vi "LJM logger write register list config.vi"(9 "Register List":string[](array[string])=["DAC0", "DAC1"], 10 "Filename":string="LJM_Open_Any.cfg", 11 "Working Directory":path) -> (0 "error out":errorcluster)   [LabVIEW 2026]
uses:
  <vilib>/Utility/config.llb/Write Key (String).vi
  <vilib>/Utility/config.llb/NI_LVConfig.lvlib
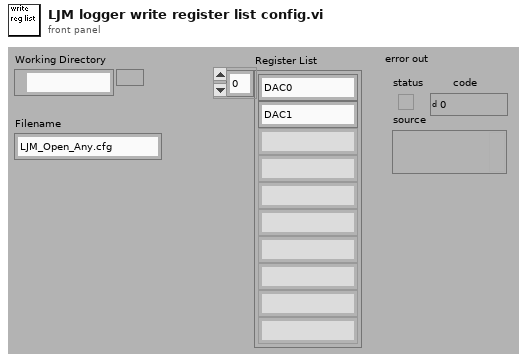
[diagram p1: front panel]
types:
  T1 = typedef "NI_LVConfig.lvlib/Config Data RefNum.ctl" = refnum<k1>
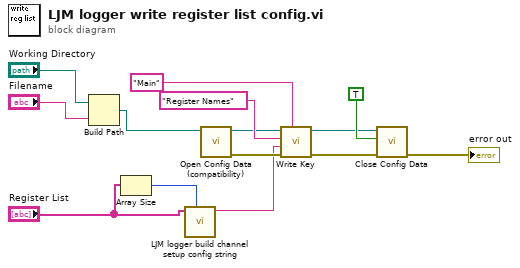
[diagram p0: block diagram]
diagram:
  n1 = Build Path(base path="Working Directory", name or relative path="Filename") -> (appended path=w12:path)
  n2 = Array Size(array="Register List") -> (size(s)=w4:i32)
  n3 = call "LJM logger build channel setup config string.vi"("Max Num Elements"=w4, "String list 1"="Register List") -> ("String 1 formatted"=w3:string)  [unwired: 6 in, 3 out]
  n4 = call <vilib>:"Open Config Data (compatibility).vi"("configuration file path"=w12) -> ("error out"=w6:errorcluster, "refnum"=w7:T1)  [unwired: 8 in, 1 out]
  n5 = call-poly <vilib>:"Write Key.vi"("section"="Main", "error in (no error)"=w6, "value"=w3, "key"="Register Names", "refnum"=w7) -> ("error out"=w1:errorcluster, "refnum out"=w2:T1)  [unwired: 4 in, 1 out]
  n6 = call <vilib>:"Close Config Data.vi"("error in (no error)"=w1, "write file if changed (T)"=TRUE ("write configuration file? (F)"), "refnum"=w2) -> ("error out"=→"error out":errorcluster)  [unwired: 7 in, 1 out]
